vi "Adjust Splitter.vi"(8 "error in":errorcluster, 9 "Show":bool, 10 "Splitter Info":T1, 11 "Manual UI in":refnum<class "Manual UI.lvclass">) -> (0 "error out":errorcluster, 3 "Manual UI out":refnum<class "Manual UI.lvclass">)   [LabVIEW 2019, in "Manual UI.lvlib" / "Manual UI.lvclass"]
doc: "This override is here so child classes can act on a show/hide event.\nPrime panel does not adjust splitters"
uses:
  Project/Manual UI.lvclass
  C:/Users/Public/Documents/Development/builds/Engine/Engine.lvlibp/Project/Engine.lvclass
  builds/Engine/Engine.lvlibp/Accessors/Read Self Q.vi
  builds/Engine/Actor Framework.lvlibp/1abvi3w/vi.lib/ActorFramework/Message Enqueuer/Enqueue.vi
  builds/Engine/Actor Framework.lvlibp/1abvi3w/vi.lib/ActorFramework/Message Enqueuer/Message Enqueuer.lvclass
  Manual UI Messages/Close Instruments Msg/Close Instruments Msg.lvclass
  Manual UI Messages/Launch Instruments Msg/Launch Instruments Msg.lvclass
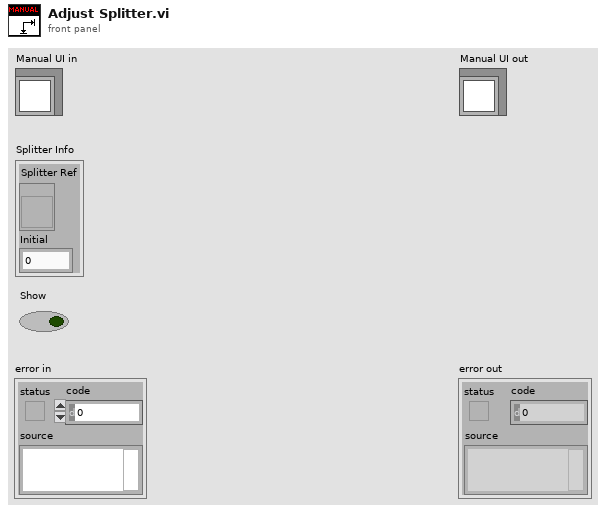
[diagram p1: front panel]
types:
  T1 = cluster{"Splitter Ref":refnum<vi>, "Initial":i32}
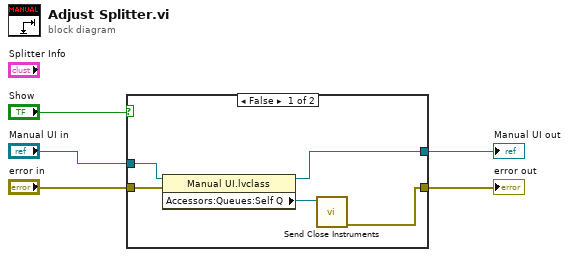
[diagram p0: block diagram]
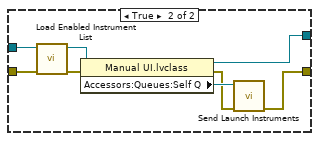
[diagram p2: hidden frame]
diagram:
  n1 = case shown="False" "Show" {
    tunnel: "Manual UI in" -> [w9 w18]
    tunnel: [w8 w14] -> w4
    tunnel: "error in" -> [w10 w17]
    tunnel: [w6 w11] -> w2
    frame False {
      n2 = property class="Manual UI.lvclass"(reference=w9, error in=w10) -> (reference out=w8:refnum<class "Manual UI.lvclass">, "Accessors:Queues:Self Q"=w7:refnum<class "Message Enqueuer.lvclass">)  [unwired: 1 out]
      n3 = call "Send Close Instruments.vi"("Message Enqueuer"=w7) -> ("error out"=w6:errorcluster)  [unwired: 9 in, 1 out]
    }
    frame True {
      n4 = call "Load Enabled Instrument List.vi"("error in"=w17, "Manual UI in"=w18) -> ("error out"=w16:errorcluster, "Manual UI out"=w15:refnum<class "Manual UI.lvclass">)  [unwired: 8 in]
      n5 = property class="Manual UI.lvclass"(reference=w15, error in=w16) -> (reference out=w14:refnum<class "Manual UI.lvclass">, error out=w12:errorcluster, "Accessors:Queues:Self Q"=w13:refnum<class "Message Enqueuer.lvclass">)
      n6 = call "Send Launch Instruments.vi"("error in (no error)"=w12, "Message Enqueuer"=w13) -> ("error out"=w11:errorcluster)  [unwired: 8 in, 1 out]
    }
  }
  "error out" <- w2
  "Manual UI out" <- w4
